vi "Get NVMEM Area Property (U32).vi"(0 "session in":refnum<k21>, 5 "NVMEM areas":refnum<k21>="$DefaultNVMEMAreas", 7 "property":refnum<k21>, 11 "error in (no error)":errorcluster) -> (4 "session out":refnum<k21>, 10 "property value":u32, 15 "error out":errorcluster)   [LabVIEW 2020, in "SLSC.lvlib"]
uses:
  <vilib>/SLSC/SLSC.lvlib
  nislsclvapi.dll
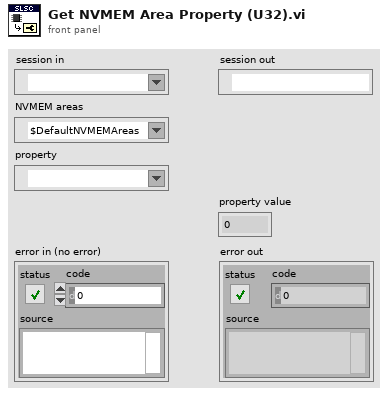
[diagram p1: front panel]
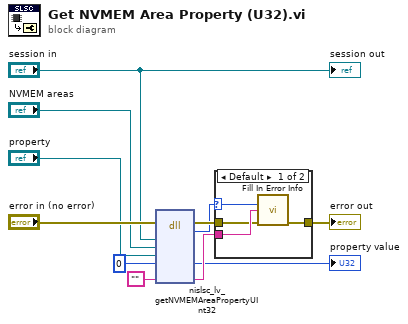
[diagram p0: block diagram]
diagram:
  n1 = dll-call lib="nislsclvapi.*" fn="nislsc_lv_getNVMEMAreaPropertyUInt32"(error in="error in (no error)", "session"="session in", "nvmemAreas"="NVMEM areas", "property"="property", "propertyValue"=u32 0, "extendedErrorInfo"="") -> (error out=w8:errorcluster, w7:i32, "propertyValue"=→"property value":u32, "extendedErrorInfo"=w9:string)  [unwired: 7 in, 1 out]
  n2 = case shown="Default" w7 {
    selector: w7 -> [w15 _]
    tunnel: w9 -> [w14 _]
    tunnel: w8 -> [w13 w16]
    tunnel: [w12 w16] -> w6
    frame Default {
      n3 = call <vilib>:"Fill In Error Info.vi"("status code"=w15, "extended error info"=w14, "error in"=w13) -> ("error out"=w12:errorcluster)  [unwired: 12 in]
    }
    frame 0 {
    }
  }
  "error out" <- w6
  "session out" <- "session in"
